vi "i2c_slave_write.vi"(5 "COM":bool, 7 "VISA name":refnum<visa-resource-name>, 9 "wLen":u16, 10 "wI2CRegAddr":u16, 11 "data":u8[](array[numeric])) -> (3 "return":i32)   [LabVIEW 2016]
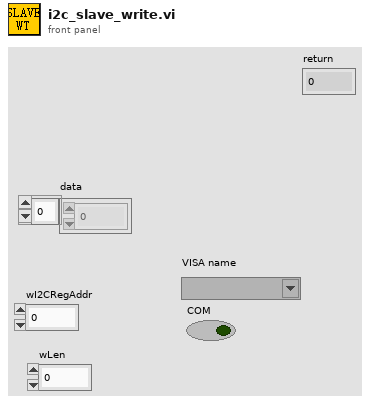
[diagram p1: front panel]
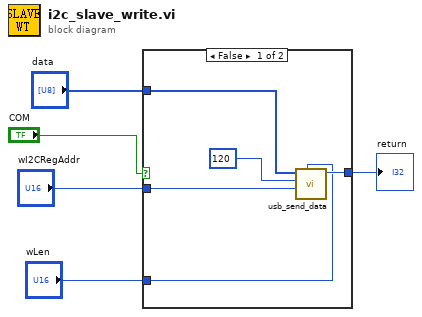
[diagram p0: block diagram]
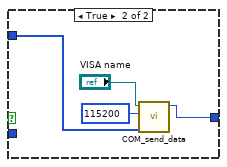
[diagram p2: hidden frame]
diagram:
  n1 = case shown="False" "COM" {
    tunnel: "data" -> [w10 w12]
    tunnel: "wI2CRegAddr" -> [w9 _]
    tunnel: "wLen" -> [w6 _]
    tunnel: [w7 w11] -> w2
    frame False {
      n2 = call "usb_send_data.vi"("byVdCmdHeaderLen"=w6, "I2C_VD_BUFFER_RW"=w9, "I2C_SLAVE_ID"=u8 120, "data"=w10) -> ("return"=w7:i32)  [unwired: 6 in, 1 out]
    }
    frame True {
      n3 = call "COM_send_data.vi"("data"=w12, "baud rate (9600)"=u32 115200, "VISA name"="VISA name") -> ("return"=w11:i32)  [unwired: 8 in]
    }
  }
  "return" <- w2
